vi "Acquire Data.vi"(8 "error in (no error)":errorcluster, 10 "Acquire Data":bool, 11 "Abstract in":refnum<class "Abstract.lvclass">) -> (0 "error out":errorcluster, 1 "Humidity Data":T1, 2 "Temp Data":T2, 3 "Abstract out":refnum<class "Abstract.lvclass">)   [LabVIEW 2021, in "Environment Chamber.lvlib" / "Abstract.lvclass"]
uses:
  Abstract.lvclass
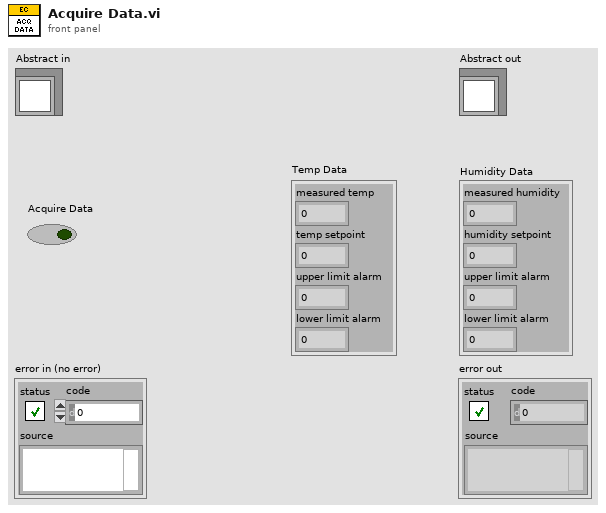
[diagram p1: front panel]
types:
  T1 = cluster{"measured humidity":dbl, "humidity setpoint":dbl, "upper limit alarm":dbl, "lower limit alarm":dbl}
  T2 = cluster{"measured temp":dbl, "temp setpoint":dbl, "upper limit alarm":dbl, "lower limit alarm":dbl}
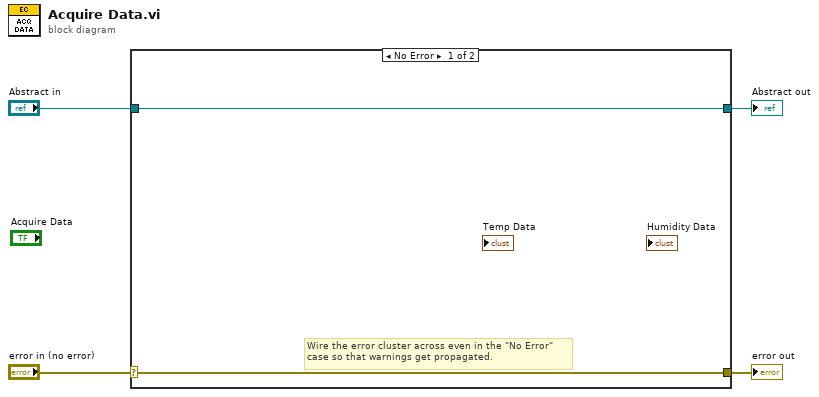
[diagram p0: block diagram]
diagram:
  n1 = case shown="No Error" "error in (no error)" {
    selector: "error in (no error)" -> [w5 w8]
    tunnel: [w5 w8] -> w3
    tunnel: [w6 w7] -> w1
    tunnel: "Abstract in" -> [w6 w7]
    frame No Error {
      # "Wire the error cluster across even in the \"No Error\"\ncase so that warnings get propagated."
    }
    frame Error {
    }
  }
  "error out" <- w3
  "Abstract out" <- w1
